vi "Virtual Axis Move.vi"(4 "Physical Axis Number (1)":u8=1 min=1, 6 "Relative To (0: virtual axis relative)":u16(ring) items=["virtual axis relative", "physical axis relative", "physical axis absolute"], 7 "Move Distance (0)":i32, 8 "error in (no error)":errorcluster, 9 "Device Number":string, 10 "Virtual Axis Number (1)":u8=1, 11 "VISA resource name":refnum<visa-resource-name>) -> (0 "error out":errorcluster, 3 "VISA resource name out":refnum<visa-resource-name>)   [LabVIEW 2018, in "Zaber A Series.lvlib"]
doc: "Moves a virtual axis. Moves can be relative to the virtual axis itself or one of the physical axes comprising it, or to an absolute position along one of the physical axes. In all cases the proportionality of relative distance moved by the physical axes will be preserved.\n\nThe move distance is specified in microstep units for the axis selected. Use the Convert Position Units to Device Units VI to convert from standard distance units.\n\nNo responses are returned with this VI, but if you would like to wait until the movement is completed to continue, you can combine this VI with the Poll Until Idle VI. \n\nThis VI requires that the Initialize VI has been called with the same serial port and that the lockstep group has been created with the Lockstep Enable VI."
uses:
  Zaber A Series.lvlib
  Private/All Commands.ctl
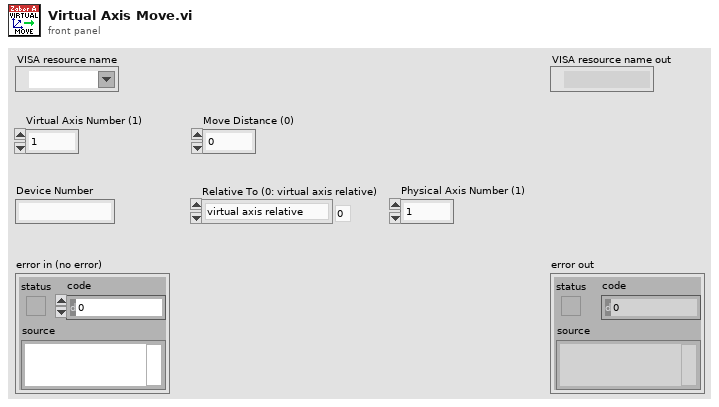
[diagram p1: front panel]
types:
  T1 = typedef "Zaber A Series.lvlib/All Commands.ctl" = string
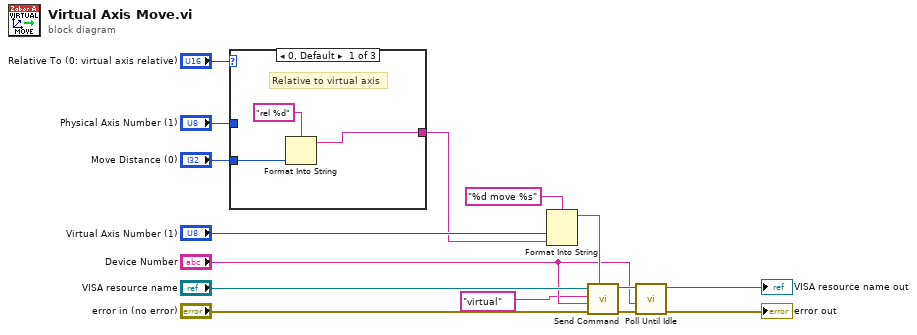
[diagram p0: block diagram]
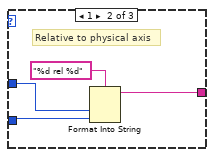
[diagram p2: hidden frame]
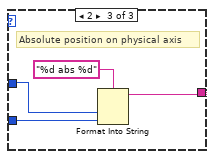
[diagram p3: hidden frame]
diagram:
  n1 = case shown="0, Default" "Relative To (0: virtual axis relative)" {
    tunnel: "Physical Axis Number (1)" -> [_ w21 w25]
    tunnel: "Move Distance (0)" -> [w17 w20 w24]
    tunnel: [w16 w19 w23] -> w4
    frame 0, Default {
      # "Relative to virtual axis"
      n2 = Format Into String(format string="rel %d", w17) -> (resulting string=w16:string)  [unwired: 2 in, 1 out]
    }
    frame 1 {
      # "Relative to physical axis"
      n3 = Format Into String(format string="%d rel %d", w21, w20) -> (resulting string=w19:string)  [unwired: 2 in, 1 out]
    }
    frame 2 {
      # "Absolute position on physical axis"
      n4 = Format Into String(format string="%d abs %d", w25, w24) -> (resulting string=w23:string)  [unwired: 2 in, 1 out]
    }
  }
  n5 = Format Into String(format string="%d move %s", "Virtual Axis Number (1)", w4) -> (resulting string=w11:string)  [unwired: 2 in, 1 out]
  n6 = call "Send Command.vi"("Data"=w11, "error in (no error)"="error in (no error)", "Device and Axis"="Device Number", "Command"=T1 "virtual" ("Complete Command List"), "VISA resource name"="VISA resource name") -> ("error out"=w9:errorcluster, "VISA resource name out"=w10:refnum<visa-resource-name>)  [unwired: 1 in, 4 out]
  n7 = call "Poll Until Idle.vi"("error in (no error)"=w9, "Device and Axis"="Device Number", "VISA resource name"=w10) -> ("error out"=→"error out":errorcluster, "VISA resource name out"=→"VISA resource name out":refnum<visa-resource-name>)  [unwired: 7 in]
